vi "Moisture_SW_Async.vi"(0 "DAQmx Physical Channel":tag, 11 "Error In":errorcluster) -> (15 "Error Out":errorcluster)   [LabVIEW 2014]
uses:
  type defs/moisture_SW_control.ctl
  <vilib>/DAQmx/create/channels.llb/DAQmx Create Channel (AO-Voltage-Basic).vi
  <vilib>/DAQmx/write.llb/DAQmx Write (Analog DBL 1Chan 1Samp).vi
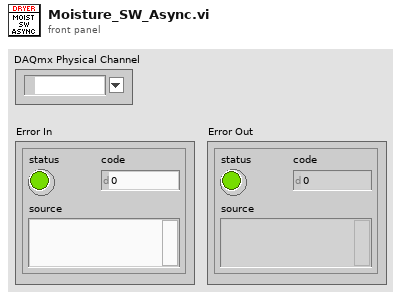
[diagram p1: front panel]
types:
  T1 = typedef "moisture_SW_control.ctl" = cluster{"State":enum16{"Stop", "Continue", "Update"}, "Data":variant}
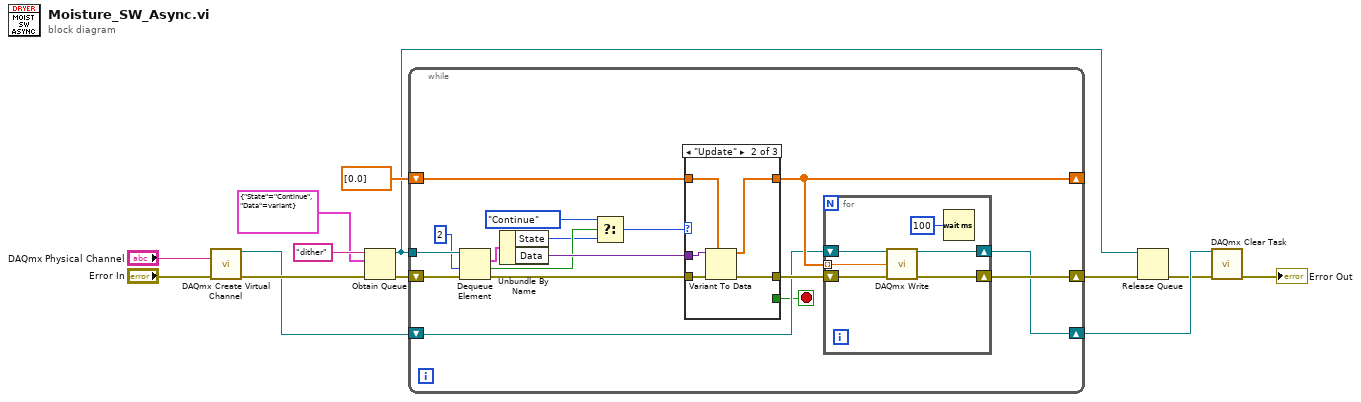
[diagram p0: block diagram]
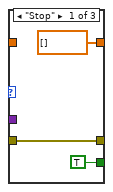
[diagram p2: hidden frame]
diagram:
  n1 = call-poly <vilib>:"DAQmx Create Virtual Channel.vi"("physical channels"="DAQmx Physical Channel", "error in"="Error In") -> ("task out"=w8:refnum<k21>, "error out"=w10:errorcluster)  [unwired: 12 in]
  n2 = Obtain Queue(name (unnamed)="dither", element data type=T1 {"State"=enum."Continue", "Data"=variant}, error in (no error)=w10) -> (queue out=w2:refnum<queue>, error out=w13:errorcluster)  [unwired: 2 in, 1 out]
  n3 = while {
    tunnel: w2 -> [w30]
    shift-right: [w21] -> _
    shift-left: dbl[] [0.0] -> [w26]
    shift-right: [w22] -> w3
    shift-left: w13 -> [w28]
    shift-right: [w14] -> w7
    shift-left: w8 -> [w20]
    stop <- w15 stop-if-true
    n4 = Dequeue Element(queue=w30, timeout in ms (-1)=2, error in (no error)=w28) -> (element=w27:T1, timed out?=w19:bool, error out=w24:errorcluster)  [unwired: 1 out]
    n5 = Unbundle By Name(w27) -> ("State"=w18:enum16{"Stop", "Continue", "Update"}, "Data"=w25:variant)
    n6 = Select(t=enum16{"Stop", "Continue", "Update"}."Continue", s=w19, f=w18) -> (s? t:f=w16:enum16{"Stop", "Continue", "Update"})
    n7 = case shown="\"Update\"" w16 {
      tunnel: w26 -> [_ w42 w45]
      tunnel: [dbl[] [] w41 w45] -> w21
      tunnel: w25 -> [_ w43 _]
      tunnel: w24 -> [w39 w44 w46]
      tunnel: [w39 w40 w46] -> w23
      tunnel: [TRUE _ _] -> w15
      frame "Stop" {
      }
      frame "Update" {
        n8 = Variant To Data(error in=w44, type=w42, Variant=w43) -> (data=w41:dbl[], error out=w40:errorcluster)
      }
      frame "Continue" {
      }
    }
    n9 = for {
      shift-right: [w35] -> w22
      shift-left: w23 -> [w36]
      tunnel: w21 -> [w34] mode=indexing
      shift-right: [w32] -> w14
      shift-left: w20 -> [w33]
      n10 = call-poly <vilib>:"DAQmx Write.vi"("task/channels in"=w33, "data"=w34, "error in"=w36) -> ("task out"=w32:refnum<k21>, "error out"=w35:errorcluster)  [unwired: 10 in, 1 out]
      n11 = Wait (ms)(milliseconds to wait=u32 100) -> ()  [unwired: 1 out]
    }
  }
  n12 = Release Queue(queue=w2, error in (no error)=w3) -> (error out=w1:errorcluster)  [unwired: 1 in, 2 out]
  n13 = call <vilib>:"DAQmx Clear Task.vi"("task in"=w7, "error in"=w1) -> ("error out"=→"Error Out":errorcluster)  [unwired: 13 in]
